vi "F Dwf Digital Uart Parity Set.vi"(8 "error in (no error)":errorcluster, 10 "parity":i32, 11 "hdwf":i32) -> (0 "error out":errorcluster, 3 "function return":i32)   [LabVIEW 2021, in "Olasdwf.lvlib"]
doc: "DWFAPI int FDwfDigitalUartParitySet(HDWF hdwf, int parity);"
uses:
  Olasdwf.lvlib
  Windows/System32/dwf.dll
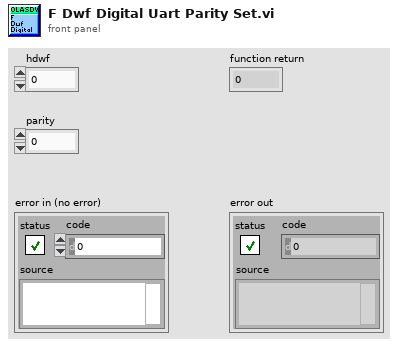
[diagram p1: front panel]
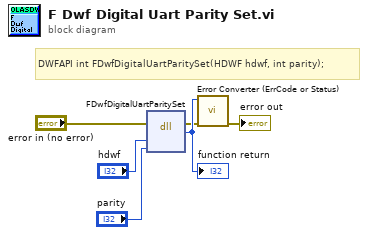
[diagram p0: block diagram]
diagram:
  # "DWFAPI int FDwfDigitalUartParitySet(HDWF hdwf, int parity);"
  n1 = dll-call lib="/Windows/System32/dwf.*" fn="FDwfDigitalUartParitySet"(error in="error in (no error)", "hdwf"="hdwf", "parity"="parity") -> (error out=w2:errorcluster, w6:i32)  [unwired: 4 in, 1 out]
  "function return" <- w6
  n2 = call "Error Converter (ErrCode or Status).vi"("error in (no error)"=w2, "error code"=w6) -> ("error out"=→"error out":errorcluster)  [unwired: 9 in]
